vi "getActorName.vi"(8 "error in":errorcluster, 9 "Actor Names":string[](array[string]), 10 "axis in":u8, 11 "connection ID":refnum<k5>) -> (0 "error out":errorcluster, 1 "ActorName out":string, 2 "axis out":u8, 3 "connection ID":refnum<k5>)   [LabVIEW 2019]
panel:
  in  "Get Command":string="com.attocube.amc.control.getActorName"
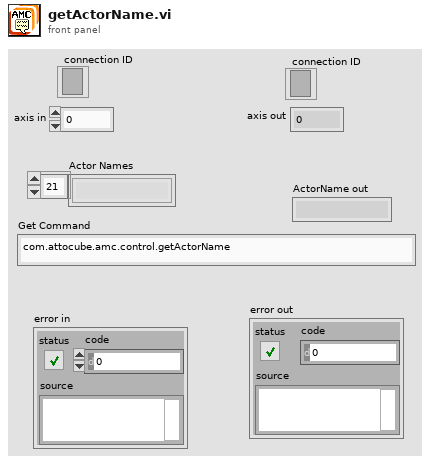
[diagram p1: front panel]
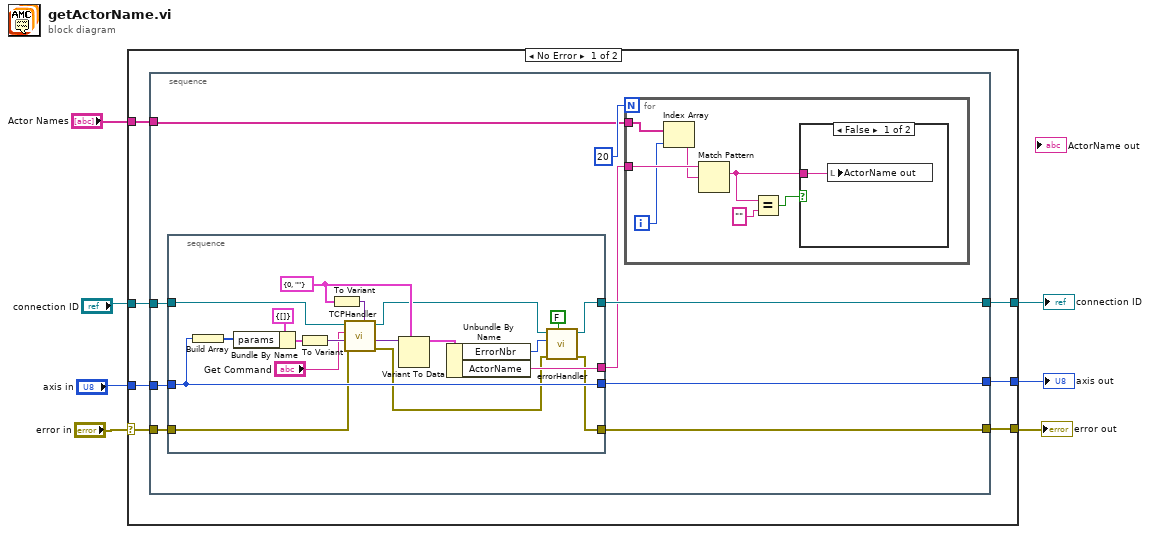
[diagram p0: block diagram]
diagram:
  n1 = case shown="No Error" "error in" {
    selector: "error in" -> [w8 w53]
    tunnel: "axis in" -> [w14 w52]
    tunnel: [w13 w53] -> w6
    tunnel: [w12 w52] -> w5
    tunnel: "connection ID" -> [w11 w51]
    tunnel: "Actor Names" -> [w10 _]
    tunnel: [w9 w51] -> w1
    frame No Error {
      n2 = stacked-sequence {
        tunnel: w14 -> [w20]
        tunnel: [w19] -> w12
        tunnel: [w17] -> w13
        tunnel: w11 -> [w16]
        tunnel: w10 -> [w22]
        tunnel: [w21] -> w9
        tunnel: w8 -> [w15]
        frame #0 {
          n3 = stacked-sequence {
            tunnel: [w30] -> w21
            tunnel: w16 -> [w35]
            tunnel: [w32] -> w18
            tunnel: w20 -> [w29]
            tunnel: [w29] -> w19
            tunnel: [w28] -> w17
            tunnel: w15 -> [w25]
            frame #0 {
              w33 = cluster{"ErrorNbr":i32, "ActorName":string} {"ErrorNbr"=0, "ActorName"=""} ("input cluster")
              n4 = Build Array(w29) -> (w39:u8[])
              n5 = Bundle By Name(cluster=cluster{"params":i16[]} {"params"=[]} ("input cluster"), "params"=w39) -> (w40:cluster{"params":i16[]})
              n6 = To Variant(anything=w40) -> (Variant=w41:variant)
              n7 = To Variant(anything=w33) -> (Variant=w34:variant)
              n8 = call <userlib>:"TCPHandler.vi"("result Types"=w34, "error in (no error)"=w25, "params"=w41, "method"="Get Command", "connection ID"=w35) -> ("error out"=w24:errorcluster, "result"=w37:variant, "connection ID"=w31:refnum<k5>)  [unwired: 3 in, 1 out]
              n9 = Variant To Data(type=w33, Variant=w37) -> (data=w42:cluster{"ErrorNbr":i32, "ActorName":string})  [unwired: 1 in, 1 out]
              n10 = Unbundle By Name(w42) -> ("ErrorNbr"=w27:i32, "ActorName"=w32:string)
              n11 = call <userlib>:"errorHandler.vi"("show popup"=FALSE, "error in"=w24, "error number"=w27, "connection ID"=w31) -> ("error out"=w28:errorcluster, "connection ID"=w30:refnum<k5>)  [unwired: 6 in]
            }
          }
          n12 = for {
            N: 20 -> [_]
            tunnel: w18 -> [w49]
            tunnel: w22 -> [w46]
            i -> [w48]
            n13 = Index Array(array=w46, index=w48) -> (element=w47:string)
            n14 = Match Pattern(string=w49, regular expression=w47) -> (match substring=w43:string)  [unwired: 1 in, 3 out]
            n15 = Equal?(x=w43, y="") -> (x = y?=w44:bool)
            n16 = case shown="False" w44 {
              tunnel: w43 -> [w50 _]
              frame False {
                n17 = local write "ActorName out"(w50) -> ()
              }
              frame True {
              }
            }
          }
        }
      }
    }
    frame Error {
    }
  }
  "error out" <- w6
  "axis out" <- w5
  "connection ID" <- w1
